vi "Toptica_UDPSearch.vi"() -> ()   [LabVIEW 2011]
panel:
  in  "name":string="192.168.1.255"
  out "FoundLasers":T1(array[cluster])
  in  "port":u16=60010
  out "net address":u32=4294967295 format="%.0x"
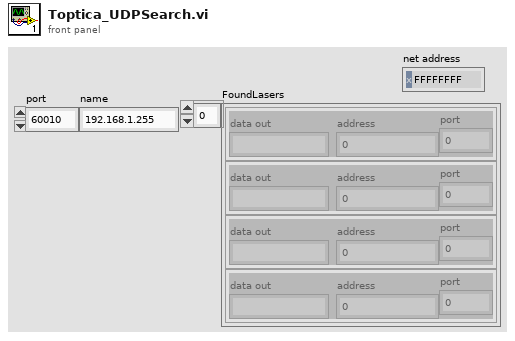
[diagram p1: front panel]
types:
  T1 = cluster{"data out":string, "address":u32, "port":u16}[]
  T2 = cluster{"data out":string, "address":u32, "port":u16}
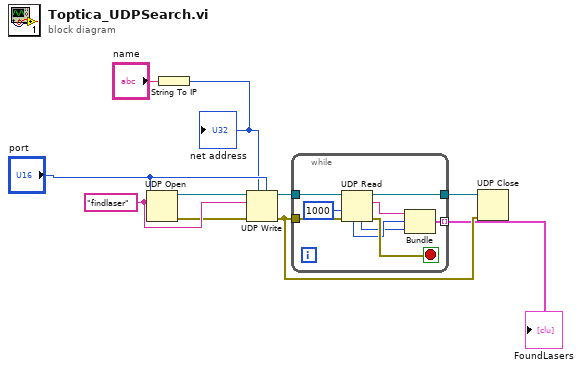
[diagram p0: block diagram]
diagram:
  w9 = "findlaser" ("service name")
  n1 = UDP Open(10:w9, 11:"port") -> (port=w10:refnum<k16>, 0:w8:errorcluster)  [unwired: 3 in, 1 out]
  n2 = String To IP(1:"name") -> (0:w1:u32)
  "net address" <- w1
  n3 = UDP Write(address=w1, port or service name="port", connection ID=w10, data in=w9, 8:w8) -> (error out=w4:errorcluster, 3:w6:refnum<k16>)  [unwired: 1 in]
  n4 = while {
    tunnel: w4 -> [w19]
    tunnel: w6 -> [w18]
    tunnel: [w15] -> w5
    tunnel: [w11] -> w3 mode=indexing
    stop <- w17 stop-if-true
    n5 = UDP Read(connection ID=w18, timeout ms (25000)=1000, 8:w19) -> (data out=w14:string, error out=w17:errorcluster, 3:w15:refnum<k16>, 4:w12:u16, 6:w13:u32)  [unwired: 1 in]
    n6 = Bundle("data out"=w14, "address"=w13, "port"=w12) -> (w11:T2)  [unwired: 1 in]
  }
  "FoundLasers" <- w3
  n7 = UDP Close(connection ID=w5, 8:w4) -> ()  [unwired: 2 out]
